vi "Registration_Create.vi"(0 "reference in":refnum<class "Registration.lvclass">, 5 "error in (no error)":errorcluster, 6 "Registration Level":T1, 7 "Application Name":string, 9 "State Queue":string[](array[string])) -> (14 "reference out":refnum<class "Registration.lvclass">, 19 "error out":errorcluster)   [LabVIEW 2022 SP3, in "Registration.lvclass"]
doc: "Constructor."
uses:
  Registration.lvclass
  C:/Program Files/National Instruments/LabVIEW 2022/vi.lib/addons/_AddQ/G#Object/G#Object.lvclass
  W:/projects/archives/23 Charette AI Group/SPWB/API/Generic Utilities_class/Generic Utilities.lvclass
  utils/Registration Type.ctl
  protected/Registration Info.ctl
  <vilib>/addons/_AddQ/G#Object/G#Object.lvclass
  Generic Utilities_class/Generic Utilities.lvclass
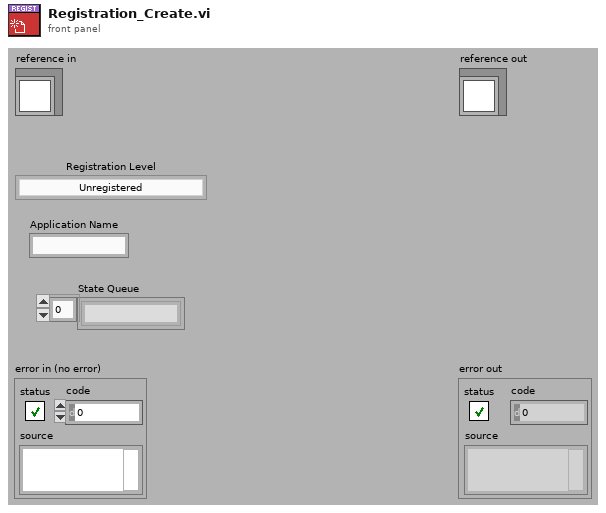
[diagram p1: front panel]
types:
  T1 = typedef "Registration.lvclass/Registration Type.ctl" = enum16{"Unregistered", "Registered - Full Activation", "Not Required- Full Activation"}
  T2 = typedef "Registration.lvclass/Registration Info.ctl" = cluster{"First Name":string, "Last Name":string, "Registration Code":string, "Registration Level":T1}
  T3 = typedef "Registration.lvclass/ObjectAttributesRef.ctl" = refnum<data-value>
  T4 = typedef "Registration.lvclass/ObjectAttributes.ctl" = cluster{"Registration Info":T2, "Object Origin":enum16{"New/Created", "Existing"}}
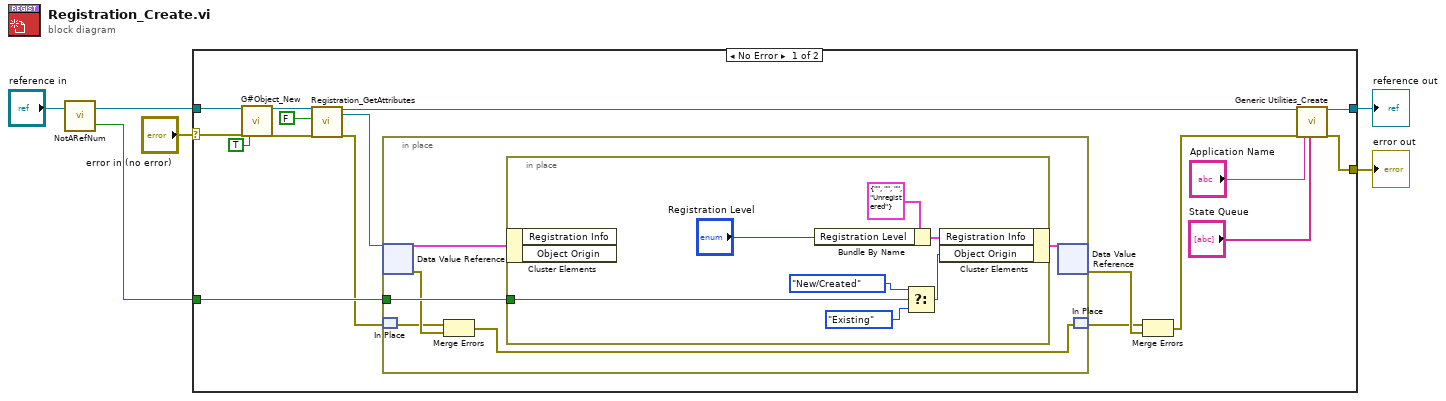
[diagram p0: block diagram]
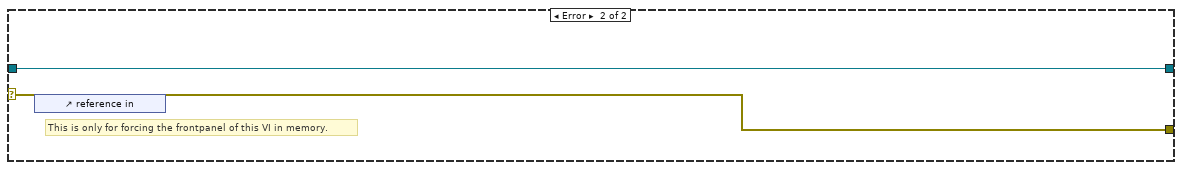
[diagram p2: hidden frame]
diagram:
  n1 = call-dynamic "NotARefNum.vi"("reference in"="reference in") -> ("not a refnum?"=w1:bool, "reference out"=w2:refnum<class "Registration.lvclass">)  [unwired: 1 in]
  n2 = case shown="No Error" "error in (no error)" {
    selector: "error in (no error)" -> [w22 w38]
    tunnel: [w12 w38] -> w5
    tunnel: [w14 w37] -> w4
    tunnel: w2 -> [w23 w37]
    tunnel: w1 -> [w9 _]
    frame No Error {
      n3 = call <vilib>:"G#Object_New.vi"("reference in"=w23, "error in (no error)"=w22, "user counter (T)?"=TRUE ("User Counter")) -> ("reference out"=w17:refnum<class "Registration.lvclass">, "error out"=w16:errorcluster)  [unwired: 14 in, 1 out]
      n4 = call "Registration_GetAttributes.vi"("reference in"=w17, "return data? (T)"=FALSE ("return data"), "error in (no error)"=w16) -> ("reference out"=w15:refnum<class "Registration.lvclass">, "attributes ref"=w19:T3, "error out"=w8:errorcluster)  [unwired: 13 in, 1 out]
      n5 = in-place {
        in-place-border: w9 -> [w27]
        n6 = in-place-dvr #1(w19) -> (w28:T4, w26:errorcluster)
        n7 = in-place-match #2(w8) -> (w25:errorcluster)
        n8 = Merge Errors(w25, w26) -> (w24:errorcluster)
        n9 = in-place {
          in-place-border: w27 -> [w30]
          n10 = in-place-cluster #3(w28) -> ()  [unwired: 2 out]
          n11 = Bundle By Name(cluster=T2 {"First Name"="", "Last Name"="", "Registration Code"="", "Registration Level"=enum."Unregistered"} ("Registration Info"), "Registration Level"="Registration Level") -> (w32:T2)
          n12 = Select(t=enum16{"New/Created", "Existing"}."New/Created" ("Object Origin"), s=w30, f=enum16{"New/Created", "Existing"}."Existing" ("Object Origin")) -> (s? t:f=w34:enum16{"New/Created", "Existing"})
          n13 = in-place-cluster #3("Registration Info"=w32, "Object Origin"=w34) -> (w29:T4)
        }
        n14 = in-place-dvr #1(w29) -> (w20:errorcluster)  [unwired: 1 out]
        n15 = in-place-match #2(w24) -> (w7:errorcluster)
      }
      n16 = Merge Errors(w7, w20) -> (w13:errorcluster)
      n17 = call "Generic Utilities_Create.vi"("reference in"=w15, "error in (no error)"=w13, "Application Name"="Application Name", "State Queue"="State Queue") -> ("reference out"=w14:refnum<class "Registration.lvclass">, "error out"=w12:errorcluster)  [unwired: 14 in]
    }
    frame Error {
      # "This is only for forcing the frontpanel of this VI in memory."
      n18 = control-ref of="reference in"() -> ()  [unwired: 1 out]
    }
  }
  "error out" <- w5
  "reference out" <- w4
